vi "例6-3.vi"() -> ()   [LabVIEW 2019]
uses:
  <vilib>/measure/NI_MABase.lvlib
panel:
  in  "停止":bool
  in  "信号类型":u16(ring) items=["正弦波", "三角波", "方波", "锯齿波"]
  in  "采样点数":dbl=1000.0
  in  "采样频率":dbl=1000.0
  in  "方波占空比":dbl=50.0
  in  "初始相位":dbl
  in  "信号幅度":dbl=1.0
  in  "信号频率":dbl=5.0
  out "波形图":waveform(dbl)(graph)
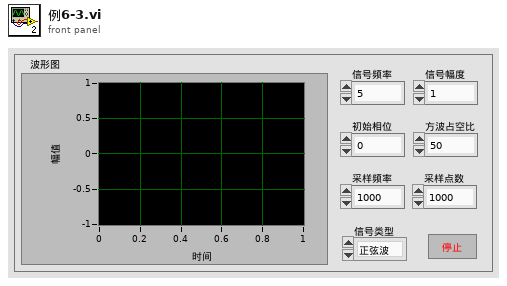
[diagram p1: front panel]
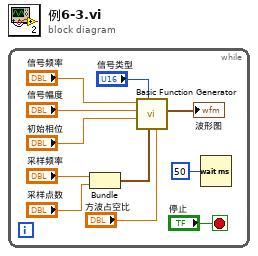
[diagram p0: block diagram]
diagram:
  n1 = while {
    stop <- "停止" stop-if-true
    n2 = Bundle("采样频率"="采样频率", "采样点数"="采样点数") -> (w9:cluster{"采样频率":dbl, "采样点数":dbl})  [unwired: 1 in]
    n3 = call <vilib>:"Basic Function Generator.vi"("square wave duty cycle (%)"="方波占空比", "sampling info"=w9, "signal type"="信号类型", "phase"="初始相位", "amplitude"="信号幅度", "frequency"="信号频率") -> ("signal out"=→"波形图":waveform(dbl))  [unwired: 3 in, 2 out]
    n4 = Wait (ms)(milliseconds to wait=50) -> ()  [unwired: 1 out]
  }
